vi "PWM_FGV_main.vi"(8 "Error In":errorcluster, 10 "PWM FGV Data":T1={"frequency"=5000.0, "Duty Cycle (%)"=0.0, "Axis Enum"=enum."X-axis", "Function Enum"=enum."Shutdown"} {"Duty Cycle (%)" min=0.0 max=100.0; "frequency" format="%_6g"}) -> (0 "Error Out":errorcluster)   [LabVIEW 2013]
doc: "This sub-VI defines the storage method for the PWM FGV, and provides the coding interface for same."
uses:
  Controls/PWM_data_cluster.ctl
  Controls/table_axis_enum.ctl
  Controls/PWM_state_enum.ctl
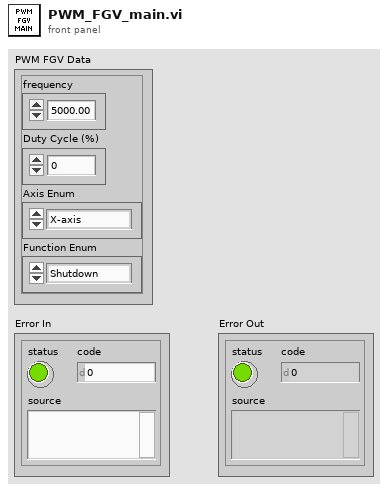
[diagram p1: front panel]
types:
  T1 = typedef "PWM_data_cluster.ctl" = cluster{"frequency":dbl, "Duty Cycle (%)":dbl, "Axis Enum":T2, "Function Enum":T3}
  T2 = typedef "table_axis_enum.ctl" = enum16{"X-axis", "Y-axis", "Z-axis", "W-axis"}
  T3 = typedef "PWM_state_enum.ctl" = enum16{"Initialize", "SetAxisSpeed", "StopAxis", "StopAll", "Shutdown"}
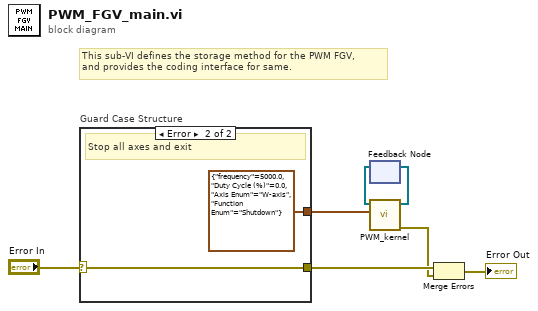
[diagram p0: block diagram]
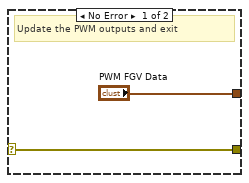
[diagram p2: hidden frame]
diagram:
  # "This sub-VI defines the storage method for the PWM FGV,\nand provides the coding interface for same."
  n1 = case "Guard Case Structure" shown="Error" "Error In" {
    selector: "Error In" -> [w9 w11]
    tunnel: [w9 w11] -> w2
    tunnel: ["PWM FGV Data" T1 {"frequency"=5000.0, "Duty Cycle (%)"=0.0, "Axis Enum"=enum."W-axis", "Function Enum"=enum."Shutdown"} ("PWM FGV Data")] -> w4
    frame No Error {
      # "Update the PWM outputs and exit"
    }
    frame Error {
      # "Stop all axes and exit"
    }
  }
  n2 = feedback #1() -> (w6:refnum<k21>[])  [unwired: 1 in]
  n3 = call "PWM_kernel.vi"("PWM FGV Data"=w4, "Task Array in"=w6) -> ("Error Out"=w1:errorcluster, "Task Array out"=w5:refnum<k21>[])  [unwired: 8 in]
  n4 = feedback-in #1(w5) -> ()
  n5 = Merge Errors(w2, w1) -> (→"Error Out":errorcluster)
